vi "Sliding Average Secondary.vi"(9 "Ln2 Filter Size":i16=10, 11 "Array In":T1=[0.0, 0.0, 0.0] format="%_6g") -> (3 "Filtered Array Out":T1 format="%_6g")   [LabVIEW 2018]
doc: "Author: Scott Hannahs <sth@magnet.fsu.edu>\nCopyright 2018 Florida State University, All rights reserved."
uses:
  SCH Data Controls/SCH Data 2 RT Array Secondary.ctl
  SCH Data Controls/SCH Data 2 RT.ctl
  SCH Data Controls/SCH Data Average Sum.ctl
  <vilib>/rvi/Memory/Memory_Emulation/nirvimemoryFastEmulation.vi
  <vilib>/rvi/Memory/Memory_Emulation/nirvimemoryEmulation.vi
  <vilib>/rvi/Emulation/niFpgaEmulationIsFPGAContextNoSignature.vi
  <vilib>/rvi/DataTransferAndStorage/Container/Common/niFpgaContainerGetUniqueNameForEmu.vi
  <vilib>/rvi/Emulation/niFpgaProcessEmulError.vi
  <vilib>/rvi/Emulation/niFpgaSctlEmulationGetInTimedLoop.vi
  <vilib>/rvi/errors/nirviReportUnexpectedCaseInternalError (U32).vi
  <vilib>/rvi/DataTransferAndStorage/Container/XNode/niFpgaContainer.xnode
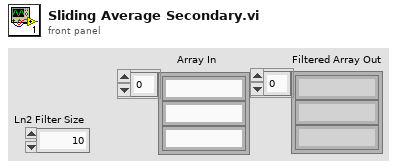
[diagram p1: front panel]
types:
  T1 = typedef "SCH Data 2 RT Array Secondary.ctl" = T2[]
  T2 = typedef "SCH Data 2 RT.ctl" = fxp<+/-,38,12>
  T3 = typedef "SCH Data Average Sum.ctl" = fxp<+/-,48,22>
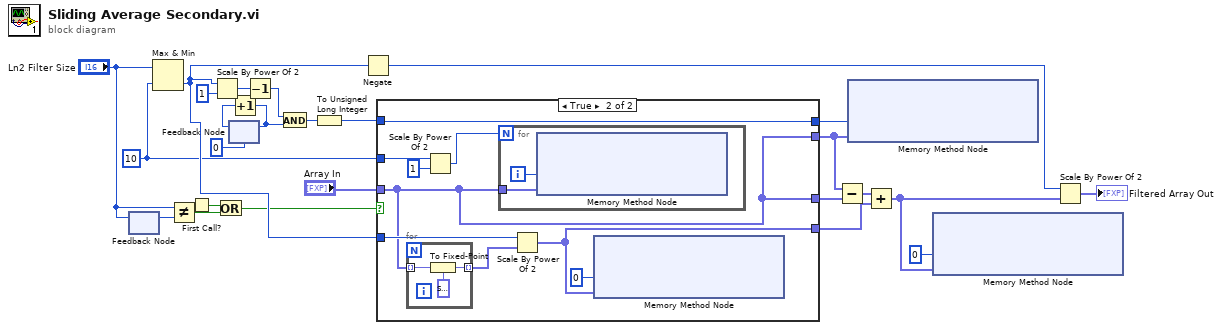
[diagram p0: block diagram]
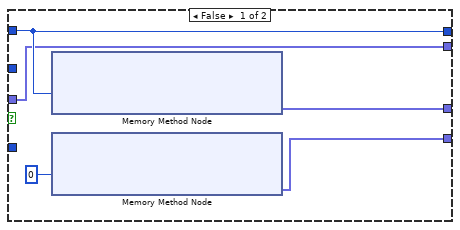
[diagram p2: hidden frame]
diagram:
  w16 = i16 10 ("y")
  n1 = feedback-in #1("Ln2 Filter Size") -> ()
  n2 = feedback #1() -> (w8:i16)  [unwired: 1 in]
  n3 = Max & Min(x="Ln2 Filter Size", y=w16) -> (min(x,y)=w22:i16)  [unwired: 1 out]
  n4 = Not Equal?(x="Ln2 Filter Size", y=w8) -> (x != y?=w6:bool)
  n5 = First Call?() -> (First Call?: T/F=w17:bool)
  n6 = Scale By Power Of 2(n=w22, x=i16 1 ("n")) -> (x*2^n=w23:i16)
  n7 = Or(x=w17, y=w6) -> (x .or. y?=w7:bool)
  n8 = feedback #2(u16 0 ("y")) -> (w3:u16)
  n9 = Increment(x=w3) -> (x+1=w1:u16)
  n10 = feedback-in #2(w1) -> ()
  n11 = Decrement(x=w23) -> (x-1=w18:i16)
  n12 = And(x=w18, y=w1) -> (x .and. y?=w25:u16)
  n13 = To Unsigned Long Integer(number=w25) -> (unsigned 32bit integer=w11:u32)
  n14 = Negate(x=w22) -> (-x=w20:i16)
  n15 = case shown="True" w7 {
    tunnel: w16 -> [_ w36]
    tunnel: [w30 w33] -> w15
    tunnel: [w29 w31] -> w14
    tunnel: w11 -> [w28 w35]
    tunnel: [w28 w35] -> w10
    tunnel: "Array In" -> [w26 w31]
    tunnel: [w26 w31] -> w4
    tunnel: w22 -> [_ w34]
    frame False {
      n16 = xnode ("Memory Method Node")("Address"=w28) -> ("Data"=w29:fxp<+/-,38,12>[])  [unwired: 1 in, 1 out]
      n17 = xnode ("Memory Method Node")("Address"=u32 0) -> ("Data"=w30:fxp<+/-,48,22>[])  [unwired: 1 in, 1 out]
    }
    frame True {
      n18 = for {
        tunnel: [w42] -> w32 mode=indexing
        tunnel: w31 -> [w40] mode=indexing
        n19 = To Fixed-Point(fixed-point type=T3 0.0 ("Numeric"), number=w40) -> (fixed-point=w42:T3)
      }
      n20 = Scale By Power Of 2(n=w36, x=i16 1 ("n")) -> (x*2^n=w37:i16)
      n21 = for {
        N: w37 -> [_]
        tunnel: w31 -> [w43]
        i -> [w44]
        n22 = xnode ("Memory Method Node")("Address"=w44, "Data"=w43) -> ()  [unwired: 1 in, 1 out]
      }
      n23 = Scale By Power Of 2(n=w34, x=w32) -> (x*2^n=w33:T3[])
      n24 = xnode ("Memory Method Node")("Address"=u32 0, "Data"=w33) -> ()  [unwired: 1 in, 1 out]
    }
  }
  n25 = Subtract(x=w4, y=w14) -> (x-y=w21:fxp<+/-,39,13>[])
  n26 = xnode ("Memory Method Node")("Address"=w10, "Data"=w4) -> ()  [unwired: 1 in, 1 out]
  n27 = Add(x=w21, y=w15) -> (x+y=w12:T3[])
  n28 = xnode ("Memory Method Node")("Address"=u32 0, "Data"=w12) -> ()  [unwired: 1 in, 1 out]
  n29 = Scale By Power Of 2(n=w20, x=w12) -> (x*2^n=→"Filtered Array Out":T3[])
